vi "Cryo Magnet (SubVI) wo checking.vi"(0 "Instrument parameters":T1, 1 "String in":refnum<vi>, 3 "Max Rate":dbl=0.5 format="%#_13g", 5 "Target":dbl, 7 "Present value":dbl, 9 "Sweep rate":dbl, 11 "error in (no error)":errorcluster, 12 "Timeout (s)":u16, 14 "Default Rate":dbl=0.25 format="%#_13g") -> (4 "Instrument parameters out":T1, 6 "Last field":dbl, 15 "error out":errorcluster)   [LabVIEW 2025]
uses:
  TYPE DEFS/S2DS_Instrument parameters.ctl
  Cryo.lvlib
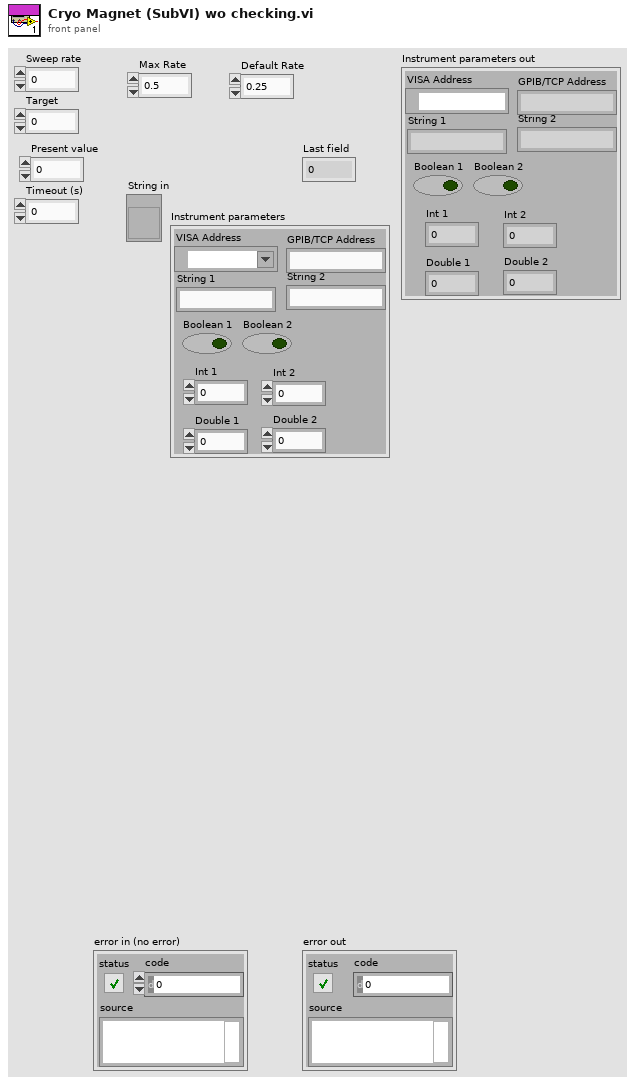
[diagram p1: front panel]
types:
  T1 = typedef "S2DS_Instrument parameters.ctl" = cluster{"VISA Address":refnum<visa-resource-name>, "GPIB/TCP Address":string, "String 1":string, "String 2":string, "Boolean 1":bool, "Boolean 2":bool, "Int 1":i32, "Int 2":i32, "Double 1":dbl, "Double 2":dbl}
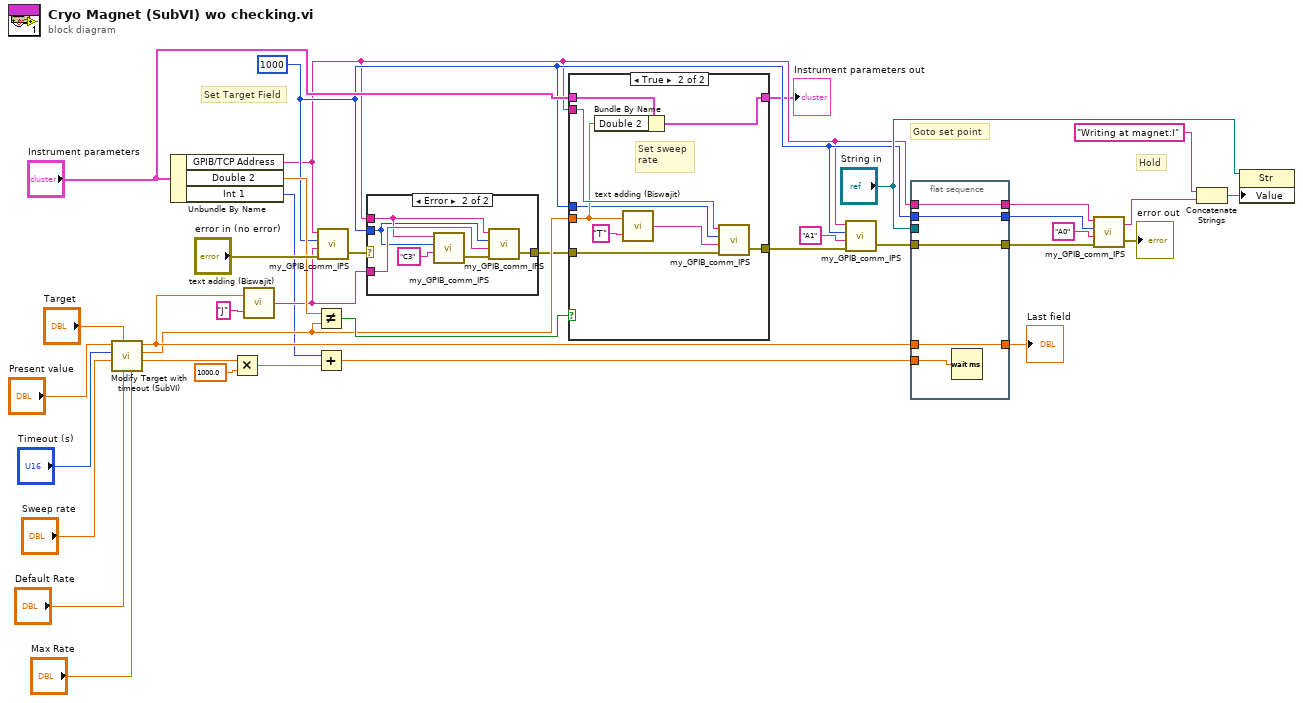
[diagram p0: block diagram]
diagram:
  w7 = u32 1000 ("Timeout (ms)")
  # "Goto set point"
  # "Set Target Field"
  # "Hold"
  n1 = call "Modify Target with timeout (SubVI).vi"("Max Rate"="Max Rate", "Default Rate"="Default Rate", "Target in"="Target", "Sweep rate in"="Sweep rate", "Timeout (s) in"="Timeout (s)", "Present value"="Present value") -> ("Timeout (s) out"=w11:dbl, "Sweep rate out"=w14:dbl, "Target out"=w16:dbl)  [unwired: 3 in]
  n2 = Unbundle By Name("Instrument parameters") -> ("GPIB/TCP Address"=w5:string, "Double 2"=w19:dbl, "Int 1"=w1:i32)
  n3 = Multiply(x=w11, y=1000.0) -> (x*y=w3:dbl)
  n4 = call "text adding (Biswajit).vi"("string"="J", "number"=w16) -> ("String"=w6:string)
  n5 = Not Equal?(x=w19, y=w14) -> (x != y?=w18:bool)
  n6 = Add(x=w1, y=w3) -> (x+y=w2:dbl)
  n7 = call "my_GPIB_comm_IPS.vi"("error in"="error in (no error)", "Command"=w6, "Timeout (ms)"=w7, "GPIB address"=w5) -> ("error out"=w9:errorcluster)  [unwired: 1 out]
  n8 = case shown="Error" w9 {
    selector: w9 -> [w38 _]
    tunnel: [w38 w39] -> w8
    tunnel: w5 -> [_ w41]
    tunnel: w7 -> [_ w40]
    tunnel: w6 -> [_ w42]
    frame No Error {
    }
    frame Error {
      n9 = call "my_GPIB_comm_IPS.vi"("Command"="C3", "Timeout (ms)"=w40, "GPIB address"=w41) -> ("error out"=w43:errorcluster)  [unwired: 1 in, 1 out]
      n10 = call "my_GPIB_comm_IPS.vi"("error in"=w43, "Command"=w42, "Timeout (ms)"=w40, "GPIB address"=w41) -> ("error out"=w39:errorcluster)  [unwired: 1 out]
    }
  }
  n11 = case shown="True" w18 {
    tunnel: w5 -> [_ w55]
    tunnel: w8 -> [w46 w54]
    tunnel: [w46 w53] -> w27
    tunnel: w14 -> [_ w49]
    tunnel: "Instrument parameters" -> [w45 w50]
    tunnel: w7 -> [_ w48]
    tunnel: [w45 w47] -> w4
    frame False {
    }
    frame True {
      # "Set sweep \nrate"
      n12 = Bundle By Name(cluster=w50, "Double 2"=w49) -> (w47:T1)
      n13 = call "text adding (Biswajit).vi"("string"="T", "number"=w49) -> ("String"=w52:string)
      n14 = call "my_GPIB_comm_IPS.vi"("error in"=w54, "Command"=w52, "Timeout (ms)"=w48, "GPIB address"=w55) -> ("error out"=w53:errorcluster)  [unwired: 1 out]
    }
  }
  "Instrument parameters out" <- w4
  n15 = call "my_GPIB_comm_IPS.vi"("error in"=w27, "Command"="A1", "Timeout (ms)"=w7, "GPIB address"=w5) -> ("error out"=w30:errorcluster)  [unwired: 1 out]
  n16 = flat-sequence {
    tunnel: [w58] -> w29
    tunnel: [w60] -> w36
    tunnel: [w59] -> w31
    tunnel: [w57] -> w21
    tunnel: "String in" -> [_]
    tunnel: w7 -> [w58]
    tunnel: w16 -> [w60]
    tunnel: w30 -> [w57]
    tunnel: w5 -> [w59]
    tunnel: w2 -> [w56]
    frame #0 {
      n17 = Wait (ms)(milliseconds to wait=w56) -> ()  [unwired: 1 out]
    }
  }
  n18 = call "my_GPIB_comm_IPS.vi"("error in"=w21, "Command"="A0", "Timeout (ms)"=w29, "GPIB address"=w31) -> ("error out"=→"error out":errorcluster, "Reply from Instrument"=w23:string)
  n19 = Concatenate Strings("Writing at magnet:I" ("string"), w23) -> (w22:string)
  n20 = property on="Property Node" class="Str"(reference="String in", "Value"=w22) -> ()  [unwired: 1 in, 2 out]
  "Last field" <- w36
